vi "Ctor.vi"(8 "error in (no error)":errorcluster, 11 "Team Config Panel in":refnum<class "Team Config Panel.lvclass">) -> (0 "error out":errorcluster, 3 "Team Config Panel out":refnum<class "Team Config Panel.lvclass">)   [LabVIEW 2020, in "SB App.lvlib" / "Team Config Panel.lvclass"]
uses:
  Team Config Panel.lvclass
  Team Index Data.ctl
  Position Enabled Data.ctl
  Update Team Data.ctl
  SquareBattle/Team/Team.lvclass
  SquareBattle/Position.ctl
  Team Config Panel.lvclass/Team Config Panel.ctl
  <vilib>/IlluminatedG/IG OOPanel/OOPanel/ArrayPanel/ArrayPanel.lvclass
  SquareBattle/SquareBattle.lvlib
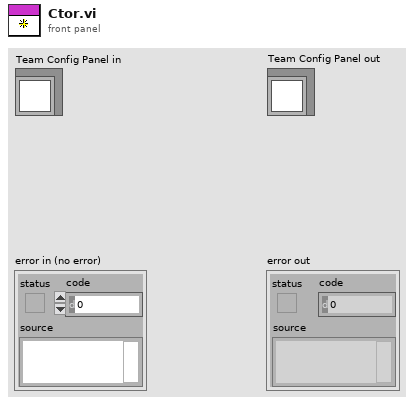
[diagram p1: front panel]
types:
  T1 = typedef "SquareBattle.lvlib/Position.ctl" = cluster{"Row":i32, "Col":i32}
  T2 = typedef "SB App.lvlib/Team Config Panel.lvclass/Update Team Data.ctl" = cluster{"Team":refnum<class "Team.lvclass">}
  T3 = typedef "SB App.lvlib/Team Config Panel.lvclass/Position Enabled Data.ctl" = cluster{"Enabled":bool}
  T4 = typedef "SB App.lvlib/Team Config Panel.lvclass/Team Index Data.ctl" = cluster{"Team Index":i32}
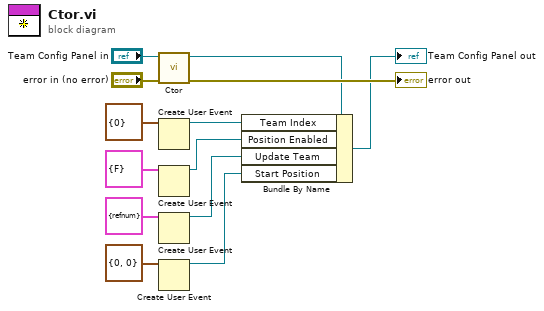
[diagram p0: block diagram]
diagram:
  n1 = call-parent "Ctor.vi"("error in (no error)"="error in (no error)", "ArrayPanel in"="Team Config Panel in") -> ("error out"=→"error out":errorcluster, "ArrayPanel out"=w8:refnum<class "Team Config Panel.lvclass">)  [unwired: 8 in]
  n2 = Create User Event(user event datatype=T4 {"Team Index"=0} ("Team Index Data")) -> (user event=w9:refnum<user-event>)  [unwired: 1 in, 1 out]
  n3 = Create User Event(user event datatype=T3 {"Enabled"=FALSE} ("Position Enabled Data")) -> (user event=w5:refnum<user-event>)  [unwired: 1 in, 1 out]
  n4 = Create User Event(user event datatype=T2 {"Team"=refnum} ("Update Team Data")) -> (user event=w3:refnum<user-event>)  [unwired: 1 in, 1 out]
  n5 = Create User Event(user event datatype=T1 {"Row"=0, "Col"=0} ("Position")) -> (user event=w1:refnum<user-event>)  [unwired: 1 in, 1 out]
  n6 = Bundle By Name(cluster=w8, "Team Index"=w9, "Position Enabled"=w5, "Update Team"=w3, "Start Position"=w1) -> (→"Team Config Panel out":refnum<class "Team Config Panel.lvclass">)
